vi "Create Serial Input Channel CSI-2 IO x8.vi"() -> (4 "serial input csi-2 io x8":T4)   [LabVIEW 2020, in "GettingStarted_Acq_Tap_148X_FPGA.lvlib"]
uses:
  GettingStarted_Acq_Tap_148X_FPGA.lvlib
  Types/Serial Input Channel IO.ctl
  Types/Serial Input Channel IO 32b.ctl
  Types/Serial Input Channel IO 64b.ctl
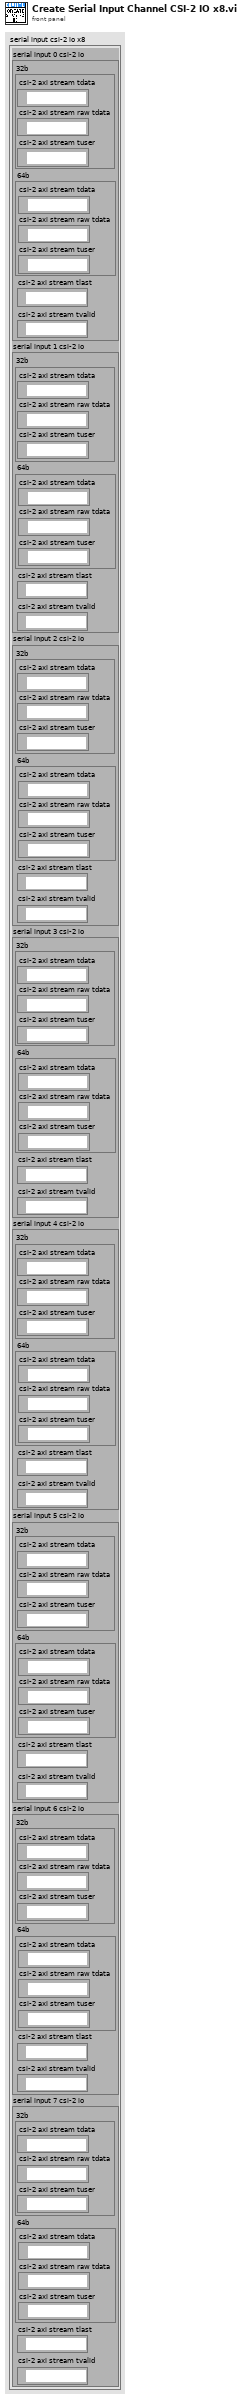
[diagram p1: front panel]
types:
  T1 = typedef "GettingStarted_Acq_Tap_148X_FPGA.lvlib/Serial Input Channel IO.ctl" = cluster{"32b":T2, "64b":T3, "csi-2 axi stream tlast":refnum<k21>, "csi-2 axi stream tvalid":refnum<k21>}
  T2 = typedef "GettingStarted_Acq_Tap_148X_FPGA.lvlib/Serial Input Channel IO 32b.ctl" = cluster{"csi-2 axi stream tdata":refnum<k21>, "csi-2 axi stream raw tdata":refnum<k21>, "csi-2 axi stream tuser":refnum<k21>}
  T3 = typedef "GettingStarted_Acq_Tap_148X_FPGA.lvlib/Serial Input Channel IO 64b.ctl" = cluster{"csi-2 axi stream tdata":refnum<k21>, "csi-2 axi stream raw tdata":refnum<k21>, "csi-2 axi stream tuser":refnum<k21>}
  T4 = cluster{"serial input 0 csi-2 io":T1, "serial input 1 csi-2 io":T1, "serial input 2 csi-2 io":T1, "serial input 3 csi-2 io":T1, "serial input 4 csi-2 io":T1, "serial input 5 csi-2 io":T1, "serial input 6 csi-2 io":T1, "serial input 7 csi-2 io":T1}
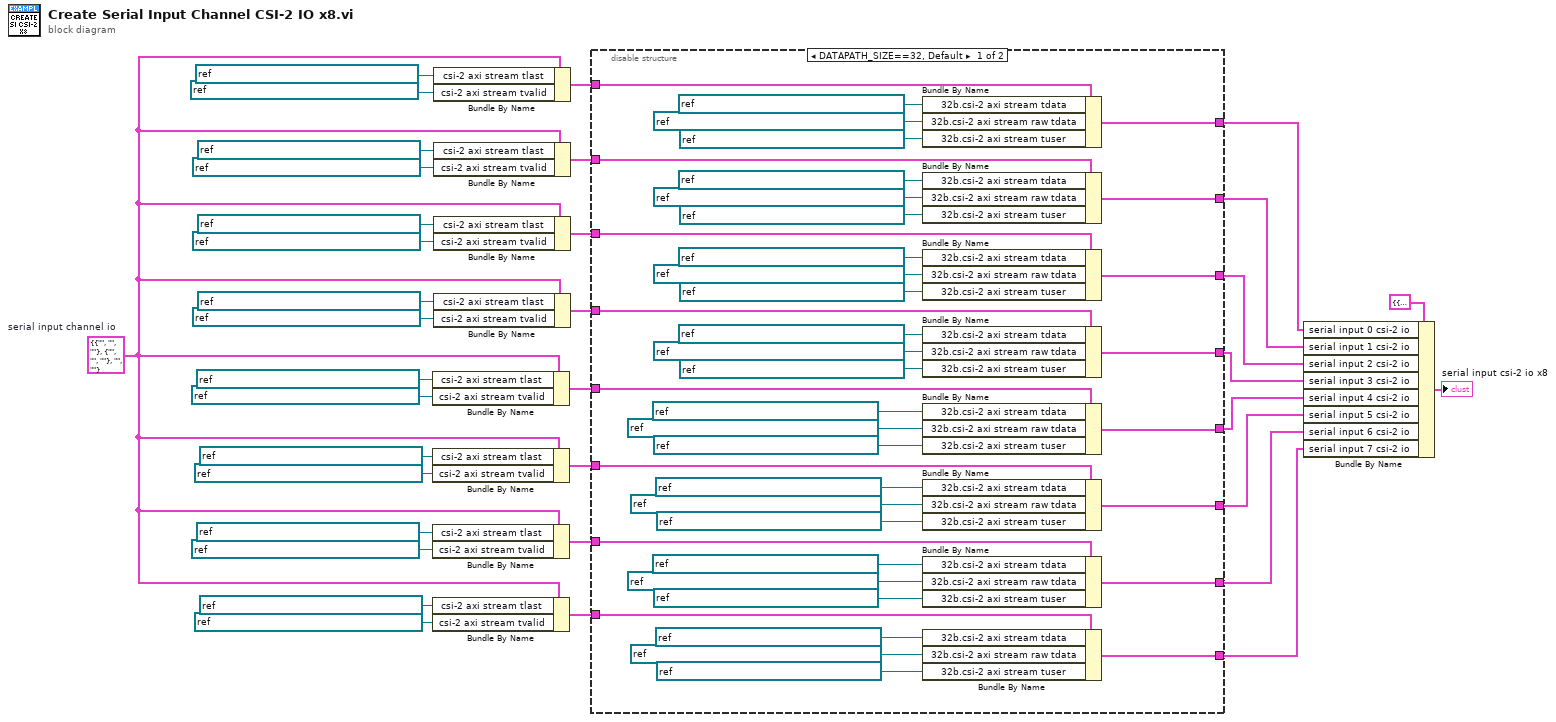
[diagram p0: block diagram]
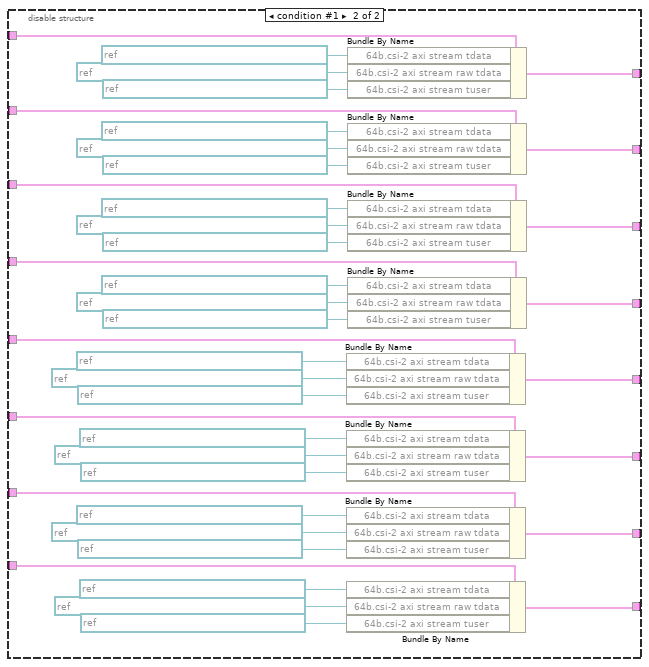
[diagram p2: hidden frame]
diagram:
  w1 = T1 {"32b"={"csi-2 axi stream tdata"="", "csi-2 axi stream raw tdata"="", "csi-2 axi stream tuser"=""}, "64b"={"csi-2 axi stream tdata"="", "csi-2 axi stream raw tdata"="", "csi-2 axi stream tuser"=""}, "csi-2 axi stream tlast"="", "csi-2 axi stream tvalid"=""}  # serial input channel io
  n1 = Bundle By Name(cluster=w1, "csi-2 axi stream tlast"=refnum<k21> "IO Socket\\SI 4 CSI-2 AXI Stream TLast" ("FPGA I/O In"), "csi-2 axi stream tvalid"=refnum<k21> "IO Socket\\SI 4 CSI-2 AXI Stream TValid" ("FPGA I/O In")) -> (w9:T1)
  n2 = Bundle By Name(cluster=w1, "csi-2 axi stream tlast"=refnum<k21> "IO Socket\\SI 5 CSI-2 AXI Stream TLast" ("FPGA I/O In"), "csi-2 axi stream tvalid"=refnum<k21> "IO Socket\\SI 5 CSI-2 AXI Stream TValid" ("FPGA I/O In")) -> (w6:T1)
  n3 = Bundle By Name(cluster=w1, "csi-2 axi stream tlast"=refnum<k21> "IO Socket\\SI 6 CSI-2 AXI Stream TLast" ("FPGA I/O In"), "csi-2 axi stream tvalid"=refnum<k21> "IO Socket\\SI 6 CSI-2 AXI Stream TValid" ("FPGA I/O In")) -> (w5:T1)
  n4 = Bundle By Name(cluster=w1, "csi-2 axi stream tlast"=refnum<k21> "IO Socket\\SI 7 CSI-2 AXI Stream TLast" ("FPGA I/O In"), "csi-2 axi stream tvalid"=refnum<k21> "IO Socket\\SI 7 CSI-2 AXI Stream TValid" ("FPGA I/O In")) -> (w7:T1)
  n5 = Bundle By Name(cluster=w1, "csi-2 axi stream tlast"=refnum<k21> "IO Socket\\SI 0 CSI-2 AXI Stream TLast" ("FPGA I/O In"), "csi-2 axi stream tvalid"=refnum<k21> "IO Socket\\SI 0 CSI-2 AXI Stream TValid" ("FPGA I/O In")) -> (w25:T1)
  n6 = Bundle By Name(cluster=w1, "csi-2 axi stream tlast"=refnum<k21> "IO Socket\\SI 1 CSI-2 AXI Stream TLast" ("FPGA I/O In"), "csi-2 axi stream tvalid"=refnum<k21> "IO Socket\\SI 1 CSI-2 AXI Stream TValid" ("FPGA I/O In")) -> (w24:T1)
  n7 = Bundle By Name(cluster=w1, "csi-2 axi stream tlast"=refnum<k21> "IO Socket\\SI 2 CSI-2 AXI Stream TLast" ("FPGA I/O In"), "csi-2 axi stream tvalid"=refnum<k21> "IO Socket\\SI 2 CSI-2 AXI Stream TValid" ("FPGA I/O In")) -> (w23:T1)
  n8 = Bundle By Name(cluster=w1, "csi-2 axi stream tlast"=refnum<k21> "IO Socket\\SI 3 CSI-2 AXI Stream TLast" ("FPGA I/O In"), "csi-2 axi stream tvalid"=refnum<k21> "IO Socket\\SI 3 CSI-2 AXI Stream TValid" ("FPGA I/O In")) -> (w22:T1)
  n9 = disable-structure shown="DATAPATH_SIZE==32, Default" {
    disable-tunnel: w25 -> [w75 w113]
    disable-tunnel: w24 -> [w74 w102]
    disable-tunnel: w23 -> [w73 w101]
    disable-tunnel: w22 -> [w72 w100]
    disable-tunnel: [w59 w99] -> w11
    disable-tunnel: [w58 w98] -> w10
    disable-tunnel: [w57 w97] -> w12
    disable-tunnel: [w56 w96] -> w13
    disable-tunnel: [w55 w77] -> w8
    disable-tunnel: w9 -> [w44 w83]
    disable-tunnel: [w43 w78] -> w4
    disable-tunnel: [w42 w79] -> w3
    disable-tunnel: [w41 w80] -> w2
    disable-tunnel: w7 -> [w40 w86]
    disable-tunnel: w6 -> [w39 w84]
    disable-tunnel: w5 -> [w38 w85]
    frame condition #0 (active) {
      n10 = Bundle By Name(cluster=w75, "32b.csi-2 axi stream tdata"=refnum<k21> "IO Socket\\SI 0 CSI-2 AXI Stream TData" ("FPGA I/O In"), "32b.csi-2 axi stream raw tdata"=refnum<k21> "IO Socket\\SI 0 CSI-2 AXI Stream Raw TData" ("FPGA I/O In"), "32b.csi-2 axi stream tuser"=refnum<k21> "IO Socket\\SI 0 CSI-2 AXI Stream TUser" ("FPGA I/O In")) -> (w59:T1)
      n11 = Bundle By Name(cluster=w74, "32b.csi-2 axi stream tdata"=refnum<k21> "IO Socket\\SI 1 CSI-2 AXI Stream TData" ("FPGA I/O In"), "32b.csi-2 axi stream raw tdata"=refnum<k21> "IO Socket\\SI 1 CSI-2 AXI Stream Raw TData" ("FPGA I/O In"), "32b.csi-2 axi stream tuser"=refnum<k21> "IO Socket\\SI 1 CSI-2 AXI Stream TUser" ("FPGA I/O In")) -> (w58:T1)
      n12 = Bundle By Name(cluster=w73, "32b.csi-2 axi stream tdata"=refnum<k21> "IO Socket\\SI 2 CSI-2 AXI Stream TData" ("FPGA I/O In"), "32b.csi-2 axi stream raw tdata"=refnum<k21> "IO Socket\\SI 2 CSI-2 AXI Stream Raw TData" ("FPGA I/O In"), "32b.csi-2 axi stream tuser"=refnum<k21> "IO Socket\\SI 2 CSI-2 AXI Stream TUser" ("FPGA I/O In")) -> (w57:T1)
      n13 = Bundle By Name(cluster=w72, "32b.csi-2 axi stream tdata"=refnum<k21> "IO Socket\\SI 3 CSI-2 AXI Stream TData" ("FPGA I/O In"), "32b.csi-2 axi stream raw tdata"=refnum<k21> "IO Socket\\SI 3 CSI-2 AXI Stream Raw TData" ("FPGA I/O In"), "32b.csi-2 axi stream tuser"=refnum<k21> "IO Socket\\SI 3 CSI-2 AXI Stream TUser" ("FPGA I/O In")) -> (w56:T1)
      n14 = Bundle By Name(cluster=w44, "32b.csi-2 axi stream tdata"=refnum<k21> "IO Socket\\SI 4 CSI-2 AXI Stream TData" ("FPGA I/O In"), "32b.csi-2 axi stream raw tdata"=refnum<k21> "IO Socket\\SI 4 CSI-2 AXI Stream Raw TData" ("FPGA I/O In"), "32b.csi-2 axi stream tuser"=refnum<k21> "IO Socket\\SI 4 CSI-2 AXI Stream TUser" ("FPGA I/O In")) -> (w55:T1)
      n15 = Bundle By Name(cluster=w39, "32b.csi-2 axi stream tdata"=refnum<k21> "IO Socket\\SI 5 CSI-2 AXI Stream TData" ("FPGA I/O In"), "32b.csi-2 axi stream raw tdata"=refnum<k21> "IO Socket\\SI 5 CSI-2 AXI Stream Raw TData" ("FPGA I/O In"), "32b.csi-2 axi stream tuser"=refnum<k21> "IO Socket\\SI 5 CSI-2 AXI Stream TUser" ("FPGA I/O In")) -> (w43:T1)
      n16 = Bundle By Name(cluster=w38, "32b.csi-2 axi stream tdata"=refnum<k21> "IO Socket\\SI 6 CSI-2 AXI Stream TData" ("FPGA I/O In"), "32b.csi-2 axi stream raw tdata"=refnum<k21> "IO Socket\\SI 6 CSI-2 AXI Stream Raw TData" ("FPGA I/O In"), "32b.csi-2 axi stream tuser"=refnum<k21> "IO Socket\\SI 6 CSI-2 AXI Stream TUser" ("FPGA I/O In")) -> (w42:T1)
      n17 = Bundle By Name(cluster=w40, "32b.csi-2 axi stream tdata"=refnum<k21> "IO Socket\\SI 7 CSI-2 AXI Stream TData" ("FPGA I/O In"), "32b.csi-2 axi stream raw tdata"=refnum<k21> "IO Socket\\SI 7 CSI-2 AXI Stream Raw TData" ("FPGA I/O In"), "32b.csi-2 axi stream tuser"=refnum<k21> "IO Socket\\SI 7 CSI-2 AXI Stream TUser" ("FPGA I/O In")) -> (w41:T1)
    }
    frame condition #1 {
      n18 = Bundle By Name(cluster=w83, "64b.csi-2 axi stream tdata"=refnum<k21> "IO Socket\\SI 4 CSI-2 AXI Stream TData" ("FPGA I/O In"), "64b.csi-2 axi stream raw tdata"=refnum<k21> "IO Socket\\SI 4 CSI-2 AXI Stream Raw TData" ("FPGA I/O In"), "64b.csi-2 axi stream tuser"=refnum<k21> "IO Socket\\SI 4 CSI-2 AXI Stream TUser" ("FPGA I/O In")) -> (w77:T1)
      n19 = Bundle By Name(cluster=w84, "64b.csi-2 axi stream tdata"=refnum<k21> "IO Socket\\SI 5 CSI-2 AXI Stream TData" ("FPGA I/O In"), "64b.csi-2 axi stream raw tdata"=refnum<k21> "IO Socket\\SI 5 CSI-2 AXI Stream Raw TData" ("FPGA I/O In"), "64b.csi-2 axi stream tuser"=refnum<k21> "IO Socket\\SI 5 CSI-2 AXI Stream TUser" ("FPGA I/O In")) -> (w78:T1)
      n20 = Bundle By Name(cluster=w85, "64b.csi-2 axi stream tdata"=refnum<k21> "IO Socket\\SI 6 CSI-2 AXI Stream TData" ("FPGA I/O In"), "64b.csi-2 axi stream raw tdata"=refnum<k21> "IO Socket\\SI 6 CSI-2 AXI Stream Raw TData" ("FPGA I/O In"), "64b.csi-2 axi stream tuser"=refnum<k21> "IO Socket\\SI 6 CSI-2 AXI Stream TUser" ("FPGA I/O In")) -> (w79:T1)
      n21 = Bundle By Name(cluster=w86, "64b.csi-2 axi stream tdata"=refnum<k21> "IO Socket\\SI 7 CSI-2 AXI Stream TData" ("FPGA I/O In"), "64b.csi-2 axi stream raw tdata"=refnum<k21> "IO Socket\\SI 7 CSI-2 AXI Stream Raw TData" ("FPGA I/O In"), "64b.csi-2 axi stream tuser"=refnum<k21> "IO Socket\\SI 7 CSI-2 AXI Stream TUser" ("FPGA I/O In")) -> (w80:T1)
      n22 = Bundle By Name(cluster=w113, "64b.csi-2 axi stream tdata"=refnum<k21> "IO Socket\\SI 0 CSI-2 AXI Stream TData" ("FPGA I/O In"), "64b.csi-2 axi stream raw tdata"=refnum<k21> "IO Socket\\SI 0 CSI-2 AXI Stream Raw TData" ("FPGA I/O In"), "64b.csi-2 axi stream tuser"=refnum<k21> "IO Socket\\SI 0 CSI-2 AXI Stream TUser" ("FPGA I/O In")) -> (w99:T1)
      n23 = Bundle By Name(cluster=w102, "64b.csi-2 axi stream tdata"=refnum<k21> "IO Socket\\SI 1 CSI-2 AXI Stream TData" ("FPGA I/O In"), "64b.csi-2 axi stream raw tdata"=refnum<k21> "IO Socket\\SI 1 CSI-2 AXI Stream Raw TData" ("FPGA I/O In"), "64b.csi-2 axi stream tuser"=refnum<k21> "IO Socket\\SI 1 CSI-2 AXI Stream TUser" ("FPGA I/O In")) -> (w98:T1)
      n24 = Bundle By Name(cluster=w101, "64b.csi-2 axi stream tdata"=refnum<k21> "IO Socket\\SI 2 CSI-2 AXI Stream TData" ("FPGA I/O In"), "64b.csi-2 axi stream raw tdata"=refnum<k21> "IO Socket\\SI 2 CSI-2 AXI Stream Raw TData" ("FPGA I/O In"), "64b.csi-2 axi stream tuser"=refnum<k21> "IO Socket\\SI 2 CSI-2 AXI Stream TUser" ("FPGA I/O In")) -> (w97:T1)
      n25 = Bundle By Name(cluster=w100, "64b.csi-2 axi stream tdata"=refnum<k21> "IO Socket\\SI 3 CSI-2 AXI Stream TData" ("FPGA I/O In"), "64b.csi-2 axi stream raw tdata"=refnum<k21> "IO Socket\\SI 3 CSI-2 AXI Stream Raw TData" ("FPGA I/O In"), "64b.csi-2 axi stream tuser"=refnum<k21> "IO Socket\\SI 3 CSI-2 AXI Stream TUser" ("FPGA I/O In")) -> (w96:T1)
    }
  }
  n26 = Bundle By Name(cluster=T4 {"serial input 0 csi-2 io"={"32b"={"csi-2 axi stream tdata"="", "csi-2 axi stream raw tdata"="", "csi-2 axi stream tuser"=""}, "64b"={"csi-2 axi stream tdata"="", "csi-2 axi stream raw tdata"="", "csi-2 axi stream tuser"=""}, "csi-2 axi stream tlast"="", "csi-2 axi stream tvalid"=""}, "serial input 1 csi-2 io"={"32b"={"csi-2 axi stream tdata"="", "csi-2 axi stream raw tdata"="", "csi-2 axi stream tuser"=""}, "64b"={"csi-2 axi stream tdata"="", "csi-2 axi stream raw tdata"="", "csi-2 axi stream tuser"=""}, "csi-2 axi stream tlast"="", "csi-2 axi stream tvalid"=""}, "serial input 2 csi-2 io"={"32b"={"csi-2 axi stream tdata"="", "csi-2 axi stream raw tdata"="", "csi-2 axi stream tuser"=""}, "64b"={"csi-2 axi stream tdata"="", "csi-2 axi stream raw tdata"="", "csi-2 axi stream tuser"=""}, "csi-2 axi stream tlast"="", "csi-2 axi stream tvalid"=""}, "serial input 3 csi-2 io"={"32b"={"csi-2 axi stream tdata"="", "csi-2 axi stream raw tdata"="", "csi-2 axi stream tuser"=""}, "64b"={"csi-2 axi stream tdata"="", "csi-2 axi stream raw tdata"="", "csi-2 axi stream tuser"=""}, "csi-2 axi stream tlast"="", "csi-2 axi stream tvalid"=""}, "serial input 4 csi-2 io"={"32b"={"csi-2 axi stream tdata"="", "csi-2 axi stream raw tdata"="", "csi-2 axi stream tuser"=""}, "64b"={"csi-2 axi stream tdata"="", "csi-2 axi stream raw tdata"="", "csi-2 axi stream tuser"=""}, "csi-2 axi stream tlast"="", "csi-2 axi stream tvalid"=""}, "serial input 5 csi-2 io"={"32b"={"csi-2 axi stream tdata"="", "csi-2 axi stream raw tdata"="", "csi-2 axi stream tuser"=""}, "64b"={"csi-2 axi stream tdata"="", "csi-2 axi stream raw tdata"="", "csi-2 axi stream tuser"=""}, "csi-2 axi stream tlast"="", "csi-2 axi stream tvalid"=""}, "serial input 6 csi-2 io"={"32b"={"csi-2 axi stream tdata"="", "csi-2 axi stream raw tdata"="", "csi-2 axi stream tuser"=""}, "64b"={"csi-2 axi stream tdata"="", "csi-2 axi stream raw tdata"="", "csi-2 axi stream tuser"=""}, "csi-2 axi stream tlast"="", "csi-2 axi stream tvalid"=""}, "serial input 7 csi-2 io"={"32b"={"csi-2 axi stream tdata"="", "csi-2 axi stream raw tdata"="", "csi-2 axi stream tuser"=""}, "64b"={"csi-2 axi stream tdata"="", "csi-2 axi stream raw tdata"="", "csi-2 axi stream tuser"=""}, "csi-2 axi stream tlast"="", "csi-2 axi stream tvalid"=""}}, "serial input 0 csi-2 io"=w11, "serial input 1 csi-2 io"=w10, "serial input 2 csi-2 io"=w12, "serial input 3 csi-2 io"=w13, "serial input 4 csi-2 io"=w8, "serial input 5 csi-2 io"=w4, "serial input 6 csi-2 io"=w3, "serial input 7 csi-2 io"=w2) -> (→"serial input csi-2 io x8":T4)
